vi "Load registry.vi"(8 "error in":errorcluster, 11 "Path":path) -> (0 "error out":errorcluster, 3 "Registry":T1)   [LabVIEW 2014]
uses:
  Loader/Registry.ctl
  <vilib>/xml/Load XML File.vi
  <vilib>/xml/Close Reference(Node).vi
  <vilib>/xml/NI_XML.lvlib
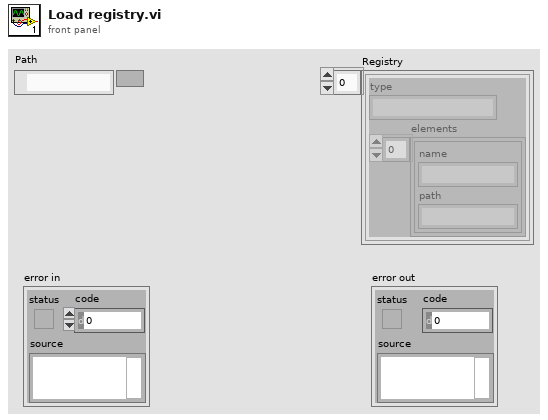
[diagram p1: front panel]
types:
  T1 = typedef "Registry.ctl" = cluster{"type":string, "elements":cluster{"name":string, "path":string}[]}[]
  T2 = cluster{"type":string, "elements":cluster{"name":string, "path":string}[]}
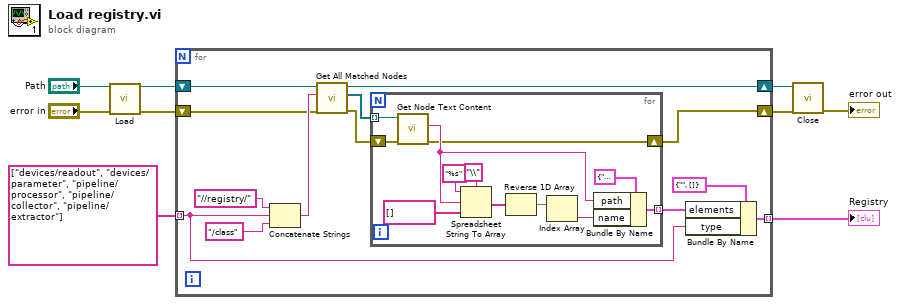
[diagram p0: block diagram]
diagram:
  n1 = call-poly <vilib>:"Load.vi"("path to XML document"="Path", "error in (no error)"="error in") -> ("DOM document out"=w7:refnum<k20>, "error out"=w4:errorcluster)  [unwired: 11 in, 1 out]
  n2 = for {
    tunnel: string[] ["devices/readout", "devices/parameter", "pipeline/processor", "pipeline/collector", "pipeline/extractor"] -> [w15] mode=indexing
    shift-right: [w17] -> w6
    shift-left: w7 -> [w18]
    tunnel: [w13] -> w5 mode=indexing
    shift-right: [w10] -> w3
    shift-left: w4 -> [w12]
    n3 = Concatenate Strings("//registry/", w15, "/class") -> (w19:string)
    n4 = call <vilib>:"Get All Matched Nodes.vi"("error in (no error)"=w12, "XPath expression"=w19, "node in"=w18) -> ("error out"=w11:errorcluster, "node result array"=w20:refnum<k20>[], "node out"=w17:refnum<k20>)  [unwired: 6 in]
    n5 = for {
      tunnel: w20 -> [w34] mode=indexing
      tunnel: [w26] -> w14 mode=indexing
      shift-right: [w23] -> w10
      shift-left: w11 -> [w24]
      n6 = call <vilib>:"Get Node Text Content.vi"("error in (no error)"=w24, "node in"=w34) -> ("error out"=w23:errorcluster, "node text"=w28:string)  [unwired: 7 in, 1 out]
      n7 = Spreadsheet String To Array(delimiter (Tab)="\\", format string="%s", spreadsheet string=w28, array type (2D Dbl)=string[] []) -> (array=w31:string[])
      n8 = Reverse 1D Array(array=w31) -> (reversed array=w30:string[])
      n9 = Index Array(array=w30) -> (element=w27:string)  [unwired: 1 in]
      n10 = Bundle By Name(cluster=cluster{"name":string, "path":string} {"name"="", "path"=""}, "path"=w28, "name"=w27) -> (w26:cluster{"name":string, "path":string})
    }
    n11 = Bundle By Name(cluster=T2 {"type"="", "elements"=[]} ("output cluster"), "elements"=w14, "type"=w15) -> (w13:T2)
  }
  "Registry" <- w5
  n12 = call-poly <vilib>:"Close.vi"("error in (no error)"=w3, "node"=w6) -> ("error out"=→"error out":errorcluster)  [unwired: 7 in]
